vi "Unflatten Value.vi"(8 "Error In":errorcluster, 10 "Value":string, 11 "StringArray In":refnum<class "1D String.lvclass">) -> (0 "Error Out":errorcluster, 3 "StringArray Out":refnum<class "1D String.lvclass">)   [LabVIEW 2017, in "Tree API.lvlib" / "1D String.lvclass"]
uses:
  1D String.lvclass
  Tree Manager/Tree.lvclass
  <vilib>/regexp/Match Regular Expression.xnode
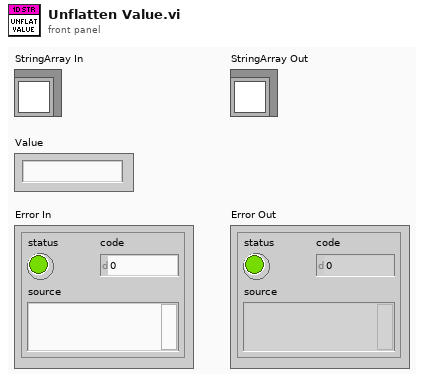
[diagram p1: front panel]
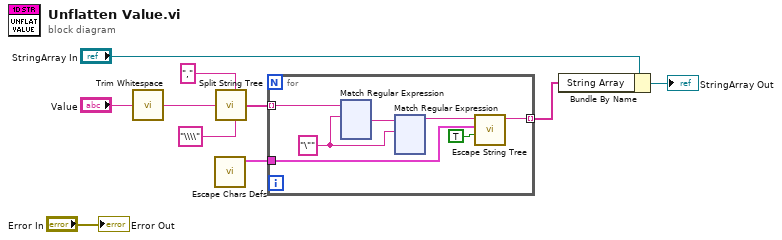
[diagram p0: block diagram]
diagram:
  n1 = call <vilib>:"Trim Whitespace.vi"("string"="Value") -> ("trimmed string"=w1:string)  [unwired: 1 in]
  n2 = call "Escape Chars Defs.vi"() -> ("Escapes"=w7:cluster{"String":string, "Escape":string}[])  [unwired: 11 in]
  n3 = call "Split String Tree.vi"("Ignore Pattern"="\\\\", "Split Pattern"=",", "Input String"=w1) -> ("Split String"=w5:string[])  [unwired: 4 in]
  n4 = for {
    tunnel: w5 -> [w14] mode=indexing
    tunnel: [w15] -> w4 mode=indexing
    tunnel: w7 -> [w17]
    w12 = "\"" ("regular expression")
    n5 = xnode "Match Regular Expression"("input string"=w14, "regular expression"=w12) -> ("after match"=w13:string)  [unwired: 4 in, 4 out]
    n6 = xnode "Match Regular Expression"("input string"=w13, "regular expression"=w12) -> ("before match"=w11:string)  [unwired: 4 in, 4 out]
    n7 = call "Escape String Tree.vi"("Reverse? (False)"=TRUE ("Remove Escapes? (False)"), "Escapes"=w17, "String In"=w11) -> ("String Out"=w15:string)  [unwired: 8 in]
  }
  n8 = Bundle By Name(cluster="StringArray In", "String Array"=w4) -> (→"StringArray Out":refnum<class "1D String.lvclass">)
  "Error Out" <- "Error In"
